vi "Recurse User Roles.vi"(8 "error in (no error)":errorcluster, 11 "Security in":refnum<class "Security.lvclass">) -> (0 "error out":errorcluster, 3 "Security out":refnum<class "Security.lvclass">)   [LabVIEW 2020, in "HTTP Server.lvlib" / "Security.lvclass"]
uses:
  Security.lvclass
  Security.lvclass/Security.ctl
  User/User.lvclass
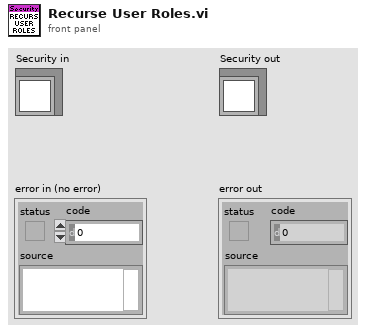
[diagram p1: front panel]
types:
  T1 = typedef "HTTP Server.lvlib/Security.lvclass/Hierarchy.ctl" = map{string, set{string}}
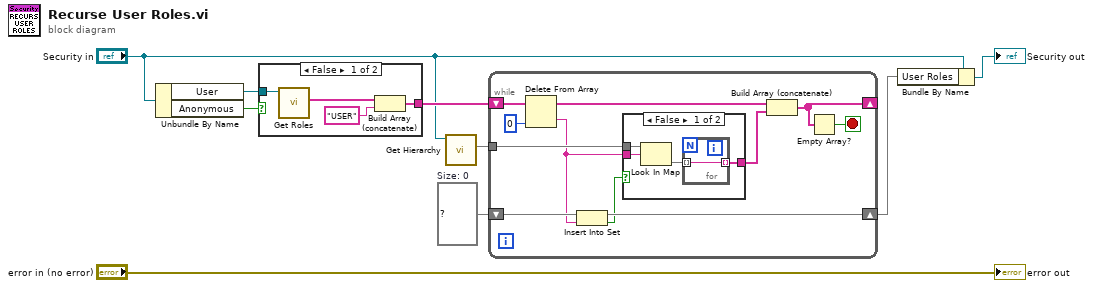
[diagram p0: block diagram]
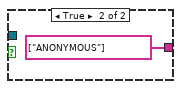
[diagram p2: hidden frame]
diagram:
  w7 = set{string} {}  # Size: 0
  n1 = Unbundle By Name("Security in") -> ("User"=w8:refnum<class "User.lvclass">, "Anonymous"=w1:bool)
  n2 = case shown="False" w1 {
    tunnel: w8 -> [w13 _]
    tunnel: [w11 string[] ["ANONYMOUS"]] -> w3
    frame False {
      n3 = call-dynamic "Get Roles.vi"("User in"=w13) -> ("Roles"=w12:string[])  [unwired: 8 in, 2 out]
      n4 = Build Array (concatenate)(w12, "USER") -> (w11:string[])
    }
    frame True {
    }
  }
  n5 = call "Get Hierarchy.vi"("Security in"="Security in") -> ("Hierarchy"=w6:T1)  [unwired: 8 in, 2 out]
  n6 = while {
    shift-right: [w16] -> _
    shift-left: w3 -> [w25]
    shift-right: [w19] -> w5
    shift-left: w7 -> [w23]
    tunnel: w6 -> [w22]
    stop <- w15 stop-if-true
    n7 = Delete From Array(array=w25, index=0) -> (deleted portion=w21:string, array with subset deleted=w20:string[])  [unwired: 1 in]
    n8 = Insert Into Set(10:w21, 11:w23) -> (2:w17:bool, 3:w19:set{string})
    n9 = case shown="False" w17 {
      tunnel: w22 -> [w29 _]
      tunnel: w21 -> [w28 _]
      tunnel: [w26 _] -> w18
      frame False {
        n10 = Look In Map(map=w29, key=w28) -> (value=w27:set{string})  [unwired: 1 in, 1 out]
        n11 = for {
          tunnel: w27 -> [w30] mode=indexing
          tunnel: [w30] -> w26 mode=indexing
        }
      }
      frame True {
      }
    }
    n12 = Build Array (concatenate)(w20, w18) -> (w16:string[])
    n13 = Empty Array?(array=w16) -> (empty?=w15:bool)
  }
  n14 = Bundle By Name(cluster="Security in", "User Roles"=w5) -> (→"Security out":refnum<class "Security.lvclass">)
  "error out" <- "error in (no error)"
